vi "Recebe resposta serial.vi"(8 "error in (no error)":errorcluster, 11 "LNA VISA resource name":refnum<visa-resource-name>) -> (0 "error out":errorcluster, 1 "timeout":bool, 2 "String Lida":string, 3 "VISA Out":refnum<visa-resource-name>)   [LabVIEW 2018]
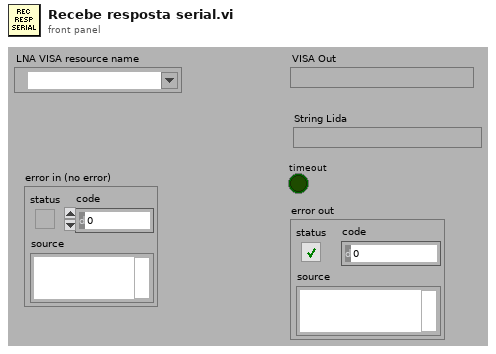
[diagram p1: front panel]
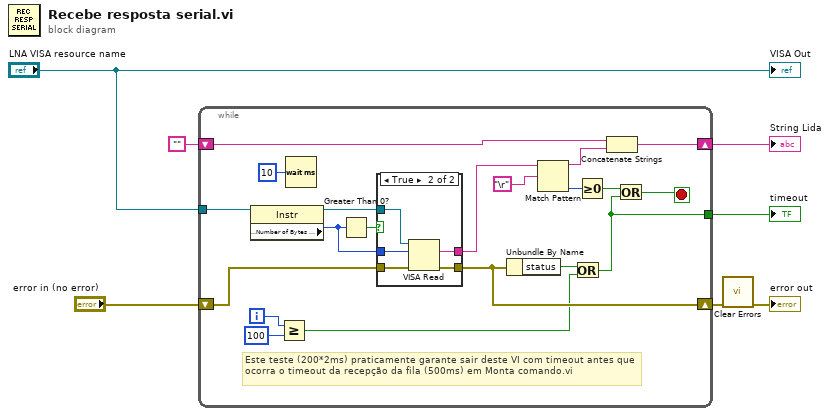
[diagram p0: block diagram]
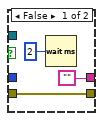
[diagram p2: hidden frame]
diagram:
  n1 = while {
    tunnel: "LNA VISA resource name" -> [w23]
    shift-right: [w26] -> w6
    shift-left: "" -> [w27]
    tunnel: [w15] -> w3
    shift-right: [w16] -> w2
    shift-left: "error in (no error)" -> [w25]
    i -> [w13]
    stop <- w24 stop-if-true
    # "Este teste (200*2ms) praticamente garante sair deste VI com timeout antes que ocorra o timeout da recepção da fila (500ms) em Monta comando.vi"
    n2 = property class="Instr"(reference=w23) -> (reference out=w22:refnum<visa-resource-name>, "Serial Settings:Number of Bytes at Serial Port"=w10:u32)  [unwired: 1 in, 1 out]
    n3 = Greater Or Equal?(x=w13, y=100) -> (x >= y?=w11:bool)
    n4 = Wait (ms)(milliseconds to wait=u32 10) -> ()  [unwired: 1 out]
    n5 = Greater Than 0?(x=w10) -> (x > 0?=w9:bool)
    n6 = case shown="True" w9 {
      tunnel: w25 -> [w29 w35]
      tunnel: w22 -> [_ w34]
      tunnel: ["" w33] -> w21
      tunnel: [w29 w32] -> w16
      tunnel: w10 -> [_ w31]
      frame False {
        n7 = Wait (ms)(milliseconds to wait=u32 2) -> ()  [unwired: 1 out]
      }
      frame True {
        n8 = VISA Read(VISA resource name=w34, byte count=w31, error in (no error)=w35) -> (read buffer=w33:string, error out=w32:errorcluster)  [unwired: 2 out]
      }
    }
    n9 = Unbundle By Name(w16) -> ("status"=w14:bool)
    n10 = Match Pattern(string=w21, regular expression="\r") -> (before substring=w19:string, offset past match=w18:i32)  [unwired: 1 in, 2 out]
    n11 = Or(x=w14, y=w11) -> (x .or. y?=w15:bool)
    n12 = Greater Or Equal To 0?(x=w18) -> (x >= 0?=w17:bool)
    n13 = Concatenate Strings(w27, w19) -> (w26:string)
    n14 = Or(x=w17, y=w15) -> (x .or. y?=w24:bool)
  }
  "String Lida" <- w6
  "timeout" <- w3
  n15 = call <vilib>:"Clear Errors.vi"("error in (no error)"=w2) -> ("error out"=→"error out":errorcluster)  [unwired: 5 in, 1 out]
  "VISA Out" <- "LNA VISA resource name"
